vi "Grabber_Mani.vi"() -> ()   [LabVIEW 2011]
uses:
  <vilib>/userdefined/High Color/IMAQdx.ctl
  CameraLan.lvclass
  <instrlib>/niHWS/nihws.llb/niHWS Open File Permissions ID.ctl
  <instrlib>/niHWS/nihws.llb/niHWS Write Analog DBL.vi
panel:
  in  "isAwake":bool
  in  "isSleeping?":bool
  in  "Magnify":bool
  in  "stop":bool
  in  "Compressor":string(combo)="DV Video Encoder"
  in  "quality":i32=-1
  in  "Rec":bool
  in  "File Path Parent Directory":path=path "C:/"
  in  "Gain":dbl(slide)=1.0 min=1.0 max=3.9810717055349722 scale=1.0..4.0
  out "acquired FPS":dbl
  out "Image":T1(plugin-control)
  in  "Session In":T2="S1019101"
  in  "Fps":i32=60
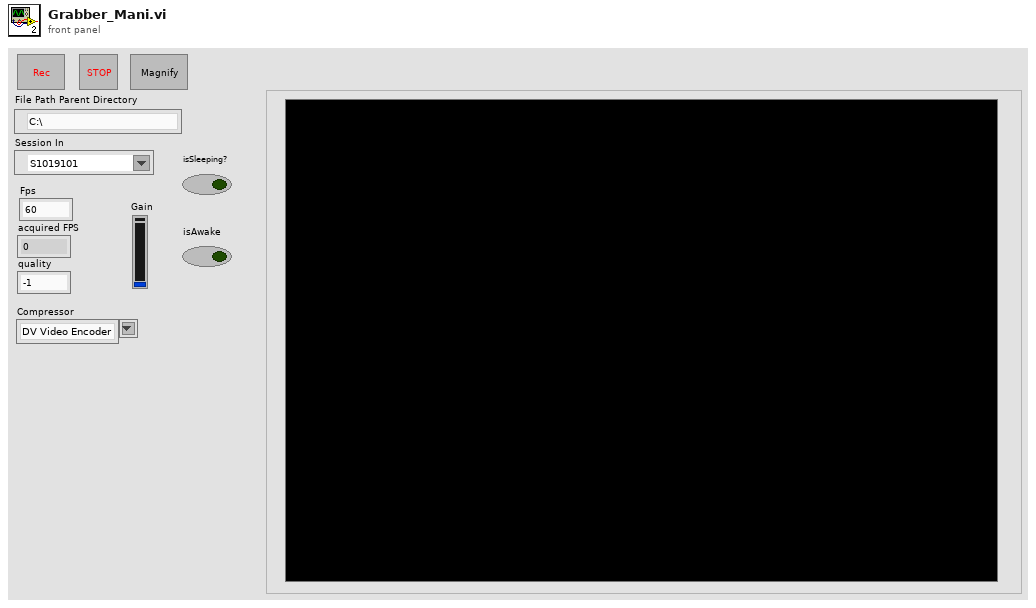
[diagram p1: front panel]
types:
  T1 = typedef "IMAQ Image.ctl" = refnum<image>
  T2 = typedef "IMAQdx.ctl" = refnum<k21>
  T3 = typedef "niHWS Open File Permissions ID.ctl" = enum32{"Read Only", "Read/Write Existing", "Read/Write/Create New", "Read/Write/Create New Always"}
  T4 = typedef "AviRefnum.ctl" = refnum<k1>
  T5 = enum32{"Invalid", "Standard", "Closed", "Hidden", "Minimized", "Maximized"}
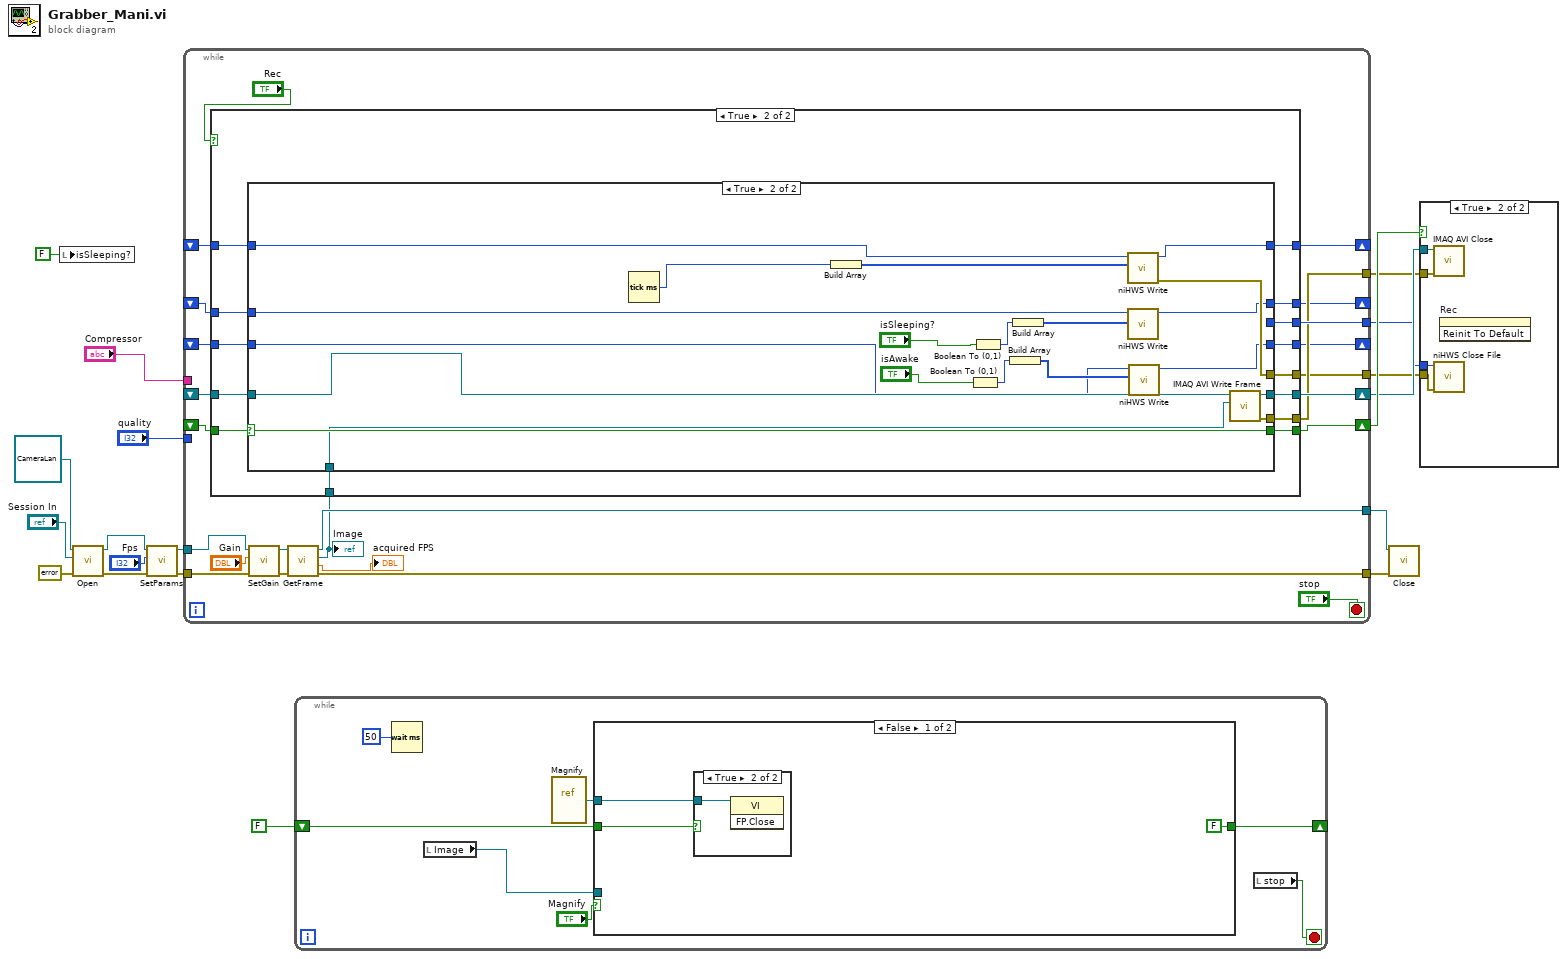
[diagram p0: block diagram]
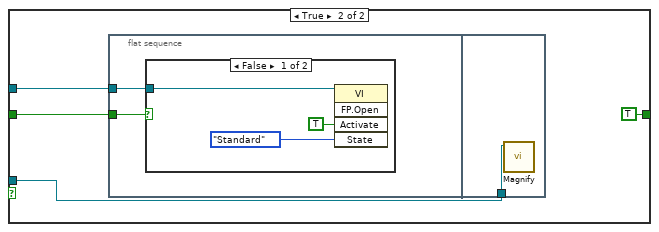
[diagram p3: hidden frame]
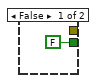
[diagram p6: hidden frame]
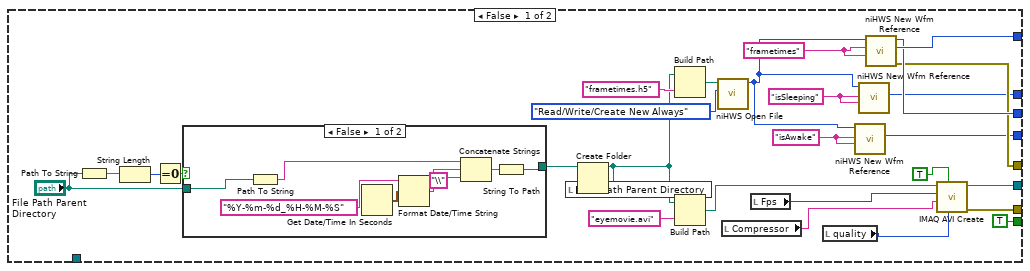
[diagram p7: hidden frame]
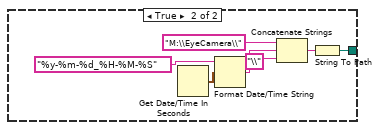
[diagram p8: hidden frame]
diagram:
  n1 = local write "isSleeping?"(FALSE ("isSleeping?")) -> ()
  n2 = call-dynamic "Open.vi"("error in (no error)"=errorcluster {"status"=FALSE, "code"=0, "source"=""}, "Session In"="Session In", "CameraLan in"=refnum<class "CameraLan.lvclass"> refnum) -> ("error out"=w14:errorcluster, "CameraLan out"=w13:refnum<class "CameraLan.lvclass">)  [unwired: 7 in]
  n3 = call-dynamic "SetParams.vi"("error in (no error)"=w14, "Fps"="Fps", "CameraLan in"=w13) -> ("error out"=w18:errorcluster, "CameraLan out"=w17:refnum<class "CameraLan.lvclass">)  [unwired: 7 in]
  n4 = while {
    tunnel: [w43] -> w16
    tunnel: w17 -> [w41]
    tunnel: w18 -> [w40]
    tunnel: [w38] -> w19
    tunnel: "Compressor" -> [_]
    tunnel: "quality" -> [_]
    shift-right: [w34] -> w7
    shift-left: _ -> [w33]
    shift-right: [w32] -> _
    shift-left: _ -> [w31]
    tunnel: [w29] -> w5
    tunnel: [w28] -> w4
    tunnel: [w27] -> w3
    shift-right: [w30] -> w6
    shift-left: _ -> [w24]
    shift-right: [w23] -> _
    shift-left: _ -> [w22]
    shift-right: [w21] -> _
    shift-left: _ -> [w20]
    stop <- "stop" stop-if-true
    n5 = call-dynamic "SetGain.vi"("error in (no error)"=w40, "Gain"="Gain", "CameraLan in"=w41) -> ("error out"=w39:errorcluster, "CameraLan out"=w42:refnum<class "CameraLan.lvclass">)  [unwired: 7 in]
    n6 = call-dynamic "GetFrame.vi"("error in (no error)"=w39, "CameraLan in"=w42) -> ("error out"=w38:errorcluster, "acquired FPS"=→"acquired FPS":dbl, "Image Out"=w25:T1, "CameraLan out"=w43:refnum<class "CameraLan.lvclass">)  [unwired: 5 in, 1 out]
    "Image" <- w25
    n7 = case shown="True" "Rec" {
      tunnel: [_ w57] -> w30
      tunnel: [_ w56] -> w28
      tunnel: [FALSE w58] -> w34
      tunnel: [_ w55] -> w32
      tunnel: w33 -> [_ w54]
      tunnel: w31 -> [_ w53]
      tunnel: [_ w52] -> w29
      tunnel: [_ w51] -> w27
      tunnel: w25 -> [_ w50]
      tunnel: w24 -> [_ w49]
      tunnel: [_ w48] -> w23
      tunnel: w22 -> [_ w47]
      tunnel: [_ w46] -> w21
      tunnel: w20 -> [_ w45]
      frame False {
      }
      frame True {
        n8 = case shown="True" w54 {
          selector: w54 -> [_ w120]
          tunnel: [TRUE w120] -> w58
          tunnel: [w82 w119] -> w57
          tunnel: [w81 w118] -> w56
          tunnel: [w66 w115] -> w55
          tunnel: w53 -> [_ w116]
          tunnel: [w65 _] -> w52
          tunnel: [w64 w114] -> w51
          tunnel: w50 -> [_ w113]
          tunnel: w49 -> [_ w112]
          tunnel: [w62 w106] -> w48
          tunnel: w47 -> [_ w107]
          tunnel: [w59 w102] -> w46
          tunnel: w45 -> [_ w101]
          frame False {
            w61 = "isAwake" ("group name (empty)")
            w63 = "isSleeping" ("group name (empty)")
            w70 = "frametimes" ("group name (empty)")
            n9 = Path To String(path="File Path Parent Directory") -> (string=w83:string)
            n10 = String Length(string=w83) -> (length=w84:i32)
            n11 = Equal To 0?(x=w84) -> (x = 0?=w74:bool)
            n12 = case shown="False" w74 {
              tunnel: [w86 w94] -> w72
              tunnel: "File Path Parent Directory" -> [w88 _]
              frame False {
                n13 = Path To String(path=w88) -> (string=w87:string)
                n14 = Get Date/Time In Seconds() -> (seconds since 1Jan1904=w93:timestamp)
                n15 = Format Date/Time String(time format string (%c)="%Y-%m-%d_%H-%M-%S", seconds (now)=w93) -> (date/time string=w91:string)  [unwired: 1 in]
                n16 = Concatenate Strings(w87, w91, "\\" ("string")) -> (w89:string)
                n17 = String To Path(string=w89) -> (path=w86:path)
              }
              frame True {
                n18 = Get Date/Time In Seconds() -> (seconds since 1Jan1904=w100:timestamp)
                n19 = Format Date/Time String(time format string (%c)="%y-%m-%d_%H-%M-%S", seconds (now)=w100) -> (date/time string=w97:string)  [unwired: 1 in]
                n20 = Concatenate Strings("M:\\EyeCamera\\", w97, "\\" ("string")) -> (w95:string)
                n21 = String To Path(string=w95) -> (path=w94:path)
              }
            }
            n22 = Create Folder(path (use dialog)=w72) -> (created path=w71:path)  [unwired: 2 in, 2 out]
            n23 = local write "File Path Parent Directory"(w71) -> ()
            n24 = Build Path(base path=w71, name or relative path="frametimes.h5" ("search string")) -> (appended path=w75:path)
            n25 = Build Path(base path=w71, name or relative path="eyemovie.avi" ("search string")) -> (appended path=w77:path)
            n26 = call <instrlib>:"niHWS Open File.vi"("permissions (0:read only)"=niHWS_Open_File_Permissions_ID."Read/Write/Create New Always", "file path"=w75) -> ("file handle"=w60:u32)  [unwired: 8 in, 1 out]
            n27 = local read "Compressor"() -> (w68:string)
            n28 = local read "Fps"() -> (w69:i32)
            n29 = local read "quality"() -> (w67:i32)
            n30 = call <instrlib>:"niHWS New Wfm Reference.vi"("waveform name (empty)"=w61, "group name (empty)"=w61, "file handle in"=w60) -> ("waveform reference"=w59:u32)  [unwired: 6 in, 2 out]
            n31 = call <instrlib>:"niHWS New Wfm Reference.vi"("waveform name (empty)"=w63, "group name (empty)"=w63, "file handle in"=w60) -> ("waveform reference"=w62:u32)  [unwired: 6 in, 2 out]
            n32 = call <instrlib>:"niHWS New Wfm Reference.vi"("waveform name (empty)"=w70, "group name (empty)"=w70, "file handle in"=w60) -> ("error out"=w64:errorcluster, "waveform reference"=w66:u32, "file handle out"=w65:u32)  [unwired: 6 in]
            n33 = call "IMAQ AVI Create"("quality"=w67, "Has Data"=TRUE, "Compression Filter"=w68, "Frames Per Second"=w69, "AVI Path"=w77) -> ("error out"=w81:errorcluster, "Avi Refnum"=w82:T4)  [unwired: 2 in, 3 out]
          }
          frame True {
            n34 = Tick Count (ms)() -> (millisecond timer value=w111:u32)
            n35 = Build Array(w111) -> (w117:u32[])
            n36 = Boolean To (0,1)(Boolean="isAwake") -> (0, 1=w105:i16)
            n37 = Boolean To (0,1)(Boolean="isSleeping?") -> (0, 1=w109:i16)
            n38 = Build Array(w105) -> (w103:i16[])
            n39 = Build Array(w109) -> (w108:i16[])
            n40 = call-poly <instrlib>:"niHWS Write.vi"("data"=w117, "waveform reference in"=w116) -> ("error out"=w114:errorcluster, "waveform reference out"=w115:u32)  [unwired: 8 in]
            n41 = call-poly <instrlib>:"niHWS Write.vi"("data"=w108, "waveform reference in"=w107) -> ("waveform reference out"=w106:u32)  [unwired: 8 in, 1 out]
            n42 = call-poly <instrlib>:"niHWS Write.vi"("data"=w103, "waveform reference in"=w101) -> ("waveform reference out"=w102:u32)  [unwired: 8 in, 1 out]
            n43 = call "IMAQ AVI Write Frame"("Image"=w113, "Avi Refnum"=w112) -> ("error out"=w118:errorcluster, "Avi Refnum (duplicate)"=w119:T4)  [unwired: 8 in]
          }
        }
      }
    }
  }
  n44 = while {
    shift-right: [w125] -> _
    shift-left: FALSE -> [w124]
    stop <- w122 stop-if-true
    n45 = Wait (ms)(milliseconds to wait=u32 50) -> ()  [unwired: 1 out]
    n46 = local read "Image"() -> (w121:T1)
    n47 = vi-ref "Magnify.vi"() -> (w127:refnum<vi>)
    n48 = case shown="False" "Magnify" {
      tunnel: w127 -> [w130 w135]
      tunnel: [FALSE TRUE] -> w125
      tunnel: w124 -> [w129 w133]
      tunnel: w121 -> [_ w132]
      frame False {
        n49 = case shown="True" w129 {
          tunnel: w130 -> [_ w131]
          frame False {
          }
          frame True {
            n50 = invoke class="VI" method="FP.Close"(reference=w131) -> ()  [unwired: 2 in, 3 out]
          }
        }
      }
      frame True {
        n51 = flat-sequence {
          tunnel: w135 -> [w137]
          tunnel: w133 -> [w136]
          tunnel: w132 -> [w141]
          frame #0 {
            n52 = case shown="False" w136 {
              tunnel: w137 -> [w139 _]
              frame False {
                n53 = invoke class="VI" method="FP.Open"(reference=w139, "Activate"=TRUE ("Wait Until Done"), "State"=T5."Standard") -> ()  [unwired: 2 in, 5 out]
              }
              frame True {
              }
            }
          }
          frame #1 {
            n54 = call "Magnify.vi"("Camera 2"=w141) -> ()  [unwired: 11 in]
          }
        }
      }
    }
    n55 = local read "stop"() -> (w122:bool)
  }
  n56 = call-dynamic "Close.vi"("error in (no error)"=w19, "CameraLan in"=w16) -> ()  [unwired: 9 in, 1 out]
  n57 = case shown="True" w7 {
    tunnel: w6 -> [_ w145]
    tunnel: w4 -> [_ w144]
    tunnel: w5 -> [_ w143]
    tunnel: w3 -> [_ w142]
    frame False {
    }
    frame True {
      n58 = call "IMAQ AVI Close"("error in (no error)"=w144, "Avi Refnum"=w145) -> ()  [unwired: 9 in, 1 out]
      n59 = call <instrlib>:"niHWS Close File.vi"("error in (no error)"=w142, "file handle"=w143) -> ()  [unwired: 9 in, 1 out]
      n60 = invoke on="Rec" class="Bool (strict)" method="Reinit To Default"() -> ()  [unwired: 3 in, 3 out]
    }
  }
